vi "configure restart stub.vi"() -> ()   [LabVIEW 2011]
panel:
  out "Command Line used to restart Spartan":string
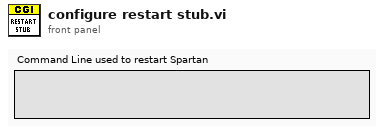
[diagram p1: front panel]
types:
  T1 = enum32{"Invalid", "Standard", "Closed", "Hidden", "Minimized", "Maximized"}
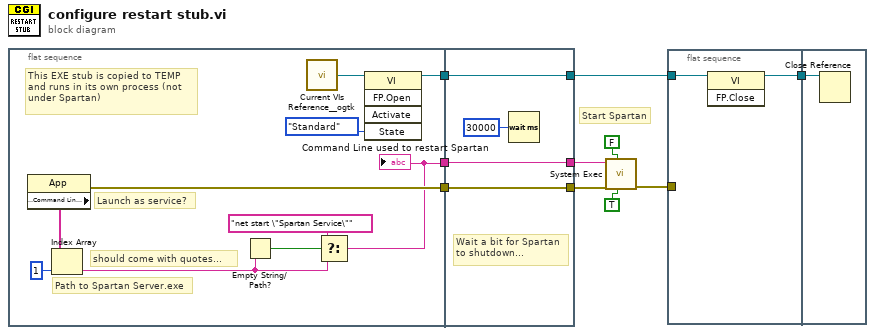
[diagram p0: block diagram]
diagram:
  # "Start Spartan"
  n1 = flat-sequence {
    tunnel: [w20] -> w3
    tunnel: [w16] -> w2
    tunnel: [w14] -> w1
    tunnel: [w22] -> w6
    tunnel: [w23] -> w4
    tunnel: [w24] -> w10
    tunnel: w3 -> [w24]
    tunnel: w2 -> [w23]
    tunnel: w1 -> [w22]
    frame #0 {
      # "This EXE stub is copied to TEMP\nand runs in its own process (not\nunder Spartan)"
      # "should come with quotes..."
      # "Launch as service?"
      # "Path to Spartan Server.exe"
      n2 = property class="App"() -> (error out=w20:errorcluster, "Application:Command Line Arguments"=w18:string[])  [unwired: 2 in, 1 out]
      n3 = Index Array(array=w18, index=1) -> (element=w11:string)
      n4 = Empty String/Path?(string/path=w11) -> (empty?=w13:bool)
      n5 = call "Current VIs Reference__ogtk.vi"() -> ("Current VI's reference"=w15:refnum<vi>)  [unwired: 5 out]
      n6 = Select(t="net start \"Spartan Service\"", s=w13, f=w11) -> (s? t:f=w16:string)
      "Command Line used to restart Spartan" <- w16
      n7 = invoke class="VI" method="FP.Open"(reference=w15, "State"=T1."Standard") -> (reference out=w14:refnum<vi>)  [unwired: 3 in, 4 out]
    }
    frame #1 {
      # "Wait a bit for Spartan\nto shutdown..."
      n8 = Wait (ms)(milliseconds to wait=u32 30000) -> ()  [unwired: 1 out]
    }
  }
  n9 = call <vilib>:"System Exec.vi"("run minimized? (F)"=TRUE, "wait until completion? (T)"=FALSE, "error in (no error)"=w10, "command line"=w4) -> ("error out"=w7:errorcluster)  [unwired: 2 in, 5 out]
  n10 = flat-sequence {
    tunnel: w7 -> [_]
    tunnel: w6 -> [w26]
    tunnel: [w25] -> w5
    tunnel: w5 -> [w27]
    frame #0 {
      n11 = invoke class="VI" method="FP.Close"(reference=w26) -> (reference out=w25:refnum<vi>)  [unwired: 2 in, 2 out]
    }
    frame #1 {
      n12 = Close Reference(reference=w27) -> ()  [unwired: 1 in, 1 out]
    }
  }
